vi "Convert Connections to UI Connections.vi"(11 "Connection List":T1[](array[typedef])) -> (3 "UI Connections List":T2[](array[typedef]))   [LabVIEW 2020, in "Routing and Faulting System Explorer.lvlib"]
uses:
  Routing and Faulting System Explorer.lvlib
  Connection Row.ctl
  Shared/Connection.ctl
  Shared/Routing and Faulting Shared.lvlib
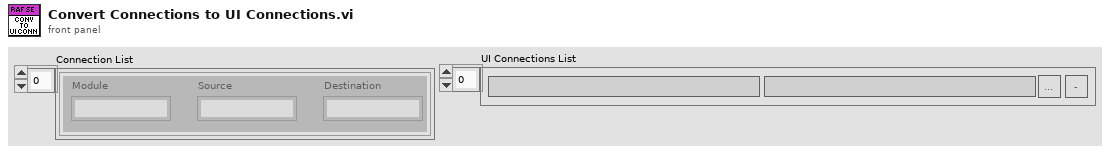
[diagram p1: front panel]
types:
  T1 = typedef "Routing and Faulting Shared.lvlib/Connection.ctl" = cluster{"Module":string, "Source":string, "Destination":string}
  T2 = typedef "Routing and Faulting System Explorer.lvlib/Connection Row.ctl" = cluster{"Source":string, "Destination":string, "Edit":bool, "Remove":bool}
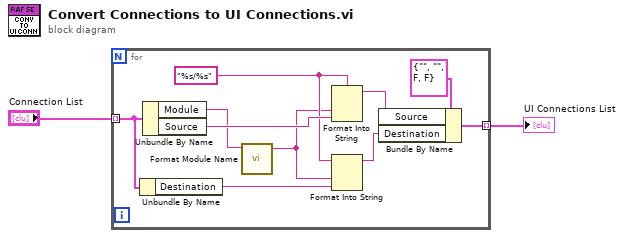
[diagram p0: block diagram]
diagram:
  n1 = for {
    tunnel: "Connection List" -> [w9] mode=indexing
    tunnel: [w5] -> w2 mode=indexing
    w10 = "%s/%s" ("format string")
    n2 = Unbundle By Name(w9) -> ("Destination"=w8:string)
    n3 = Unbundle By Name(w9) -> ("Module"=w4:string, "Source"=w11:string)
    n4 = call "Format Module Name.vi"("Module Path"=w4) -> ("Formatted Module Path"=w3:string)  [unwired: 10 in]
    n5 = Format Into String(format string=w10, w3, w11) -> (resulting string=w7:string)  [unwired: 2 in, 1 out]
    n6 = Format Into String(format string=w10, w3, w8) -> (resulting string=w6:string)  [unwired: 2 in, 1 out]
    n7 = Bundle By Name(cluster=T2 {"Source"="", "Destination"="", "Edit"=FALSE, "Remove"=FALSE} ("State and Value 2"), "Source"=w7, "Destination"=w6) -> (w5:T2)
  }
  "UI Connections List" <- w2
